vi "Попытка кнопки2.vi"() -> ()   [LabVIEW 2021]
uses:
  <vilib>/Utility/miscctls.llb/LVPositionTypeDef.ctl
  <vilib>/Utility/miscctls.llb/LVBoundsTypeDef.ctl
panel:
  in  "stop":bool
  in  "Вернуть":bool
  out "LED":bool
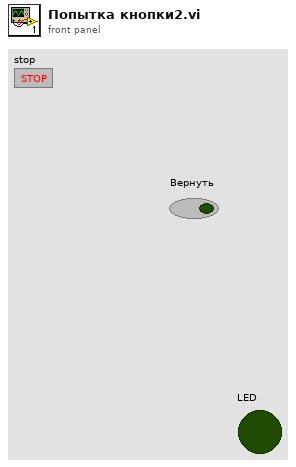
[diagram p1: front panel]
types:
  T1 = typedef "LVPositionTypeDef.ctl" = cluster{"Left":i32, "Top":i32}
  T2 = typedef "LVBoundsTypeDef.ctl" = cluster{"Width":u32, "Height":u32}
  T3 = typedef "LVPoint32TypeDef.ctl" = cluster{"Horizontal":i32, "Vertical":i32}
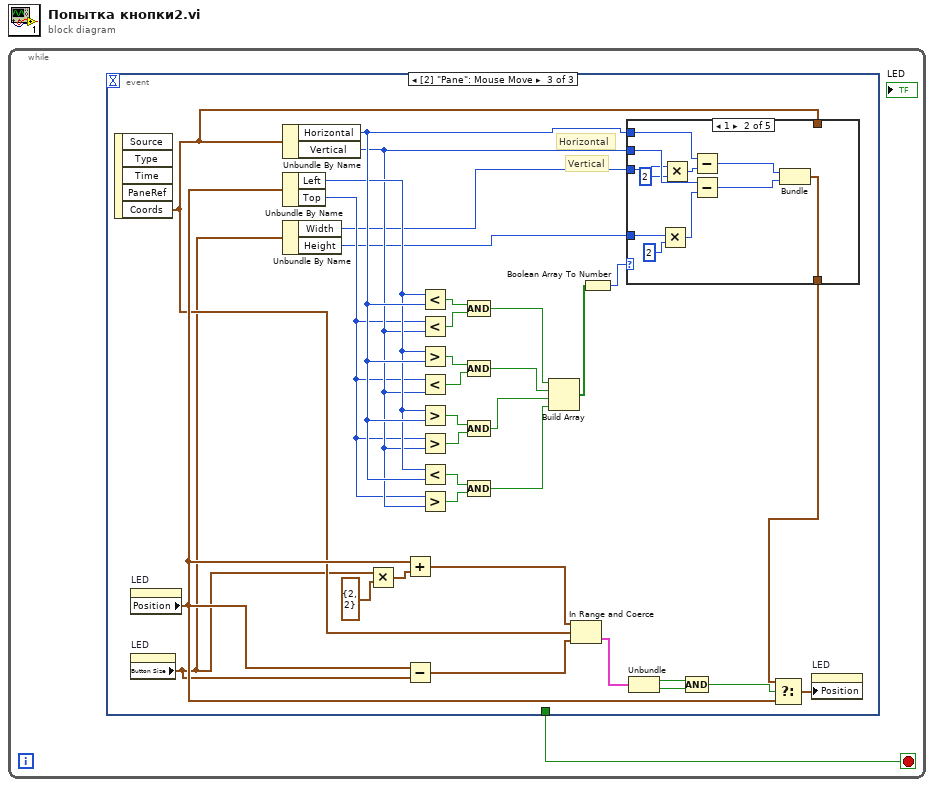
[diagram p0: block diagram]
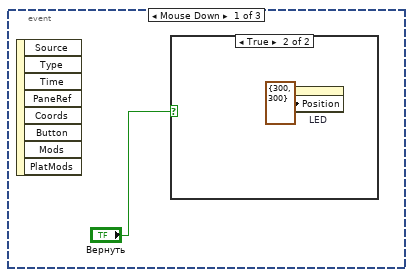
[diagram p2: hidden frame]
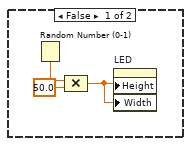
[diagram p3: hidden frame]
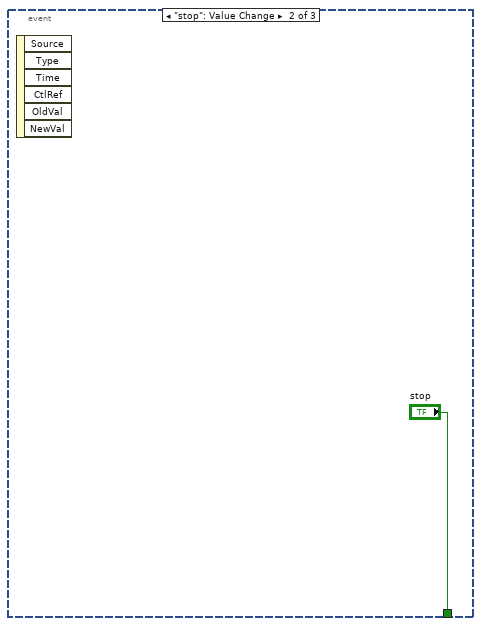
[diagram p4: hidden frame]
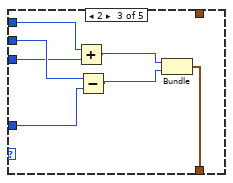
[diagram p6: hidden frame]
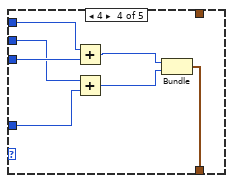
[diagram p7: hidden frame]
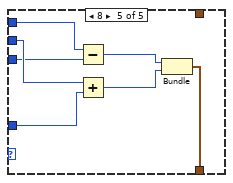
[diagram p8: hidden frame]
diagram:
  n1 = while {
    stop <- w1 stop-if-true
    n2 = event shown="[2] \"Pane\": Mouse Move" {
      selector: _ -> [_ _ _]
      dyn-events: _ -> [_ _ _]
      timeout: _ -> [_ _ _]
      tunnel: [_ "stop" _] -> w1
      event Mouse Down {
        n3 = event-data() -> ()  [unwired: 1 in, 8 out]
        n4 = case shown="True" "Вернуть" {
          frame False {
            n5 = Random Number (0-1)() -> (number: 0 to 1=w5:dbl)
            n6 = Compound Arithmetic op=MULTIPLY(w5, 50.0 ("value")) -> (w4:dbl)
            n7 = property on="LED" class="Bool (strict)"("Height"=w4, "Width"=w4) -> ()  [unwired: 2 in, 2 out]
          }
          frame True {
            n8 = property on="LED" class="Bool (strict)"("Position"=T1 {"Left"=300, "Top"=300}) -> ()  [unwired: 2 in, 2 out]
          }
        }
      }
      event "stop": Value Change {
        n9 = event-data() -> ()  [unwired: 1 in, 6 out]
      }
      event Mouse Move {
        # "Vertical"
        # "Horizontal"
        n10 = event-data() -> ("Coords"=w13:T3)  [unwired: 1 in, 4 out]
        n11 = property on="LED" class="Bool (strict)"() -> ("Position"=w33:T1)  [unwired: 2 in, 2 out]
        n12 = property on="LED" class="Bool (strict)"() -> ("Button Size"=w9:T2)  [unwired: 2 in, 2 out]
        n13 = Unbundle By Name(w13) -> ("Horizontal"=w18:i32, "Vertical"=w16:i32)
        n14 = Unbundle By Name(w33) -> ("Left"=w17:i32, "Top"=w15:i32)
        n15 = Unbundle By Name(w9) -> ("Width"=w12:u32, "Height"=w11:u32)
        n16 = Multiply(x=w9, y=T2 {"Width"=2, "Height"=2}) -> (x*y=w10:T2)
        n17 = Add(x=w33, y=w10) -> (x+y=w34:T2)
        n18 = Subtract(x=w33, y=w9) -> (x-y=w35:T2)
        n19 = Less?(x=w17, y=w18) -> (x < y?=w32:bool)
        n20 = Less?(x=w15, y=w16) -> (x < y?=w31:bool)
        n21 = Greater?(x=w17, y=w18) -> (0:w30:bool)
        n22 = Less?(x=w15, y=w16) -> (x < y?=w29:bool)
        n23 = Greater?(x=w17, y=w18) -> (0:w28:bool)
        n24 = Greater?(x=w15, y=w16) -> (0:w27:bool)
        n25 = Less?(x=w17, y=w18) -> (x < y?=w26:bool)
        n26 = Greater?(x=w15, y=w16) -> (0:w25:bool)
        n27 = Compound Arithmetic op=AND(w32, w31) -> (w24:bool)
        n28 = Compound Arithmetic op=AND(w30, w29) -> (w23:bool)
        n29 = Compound Arithmetic op=AND(w28, w27) -> (w22:bool)
        n30 = Compound Arithmetic op=AND(w26, w25) -> (w21:bool)
        n31 = Build Array(w24, w23, w22, w21) -> (w20:bool[])
        n32 = In Range and Coerce(upper limit=w34, x=w13, lower limit=w35) -> (In Range?=w38:cluster{"Width":bool, "Height":bool})  [unwired: 1 out]
        n33 = Boolean Array To Number(Boolean array=w20) -> (number=w19:u32)
        n34 = case shown="1" w19 {
          tunnel: w18 -> [_ w50 w56 w64 w68]
          tunnel: w12 -> [_ w43 w53 w63 w67]
          tunnel: w16 -> [_ w48 w55 w61 w71]
          tunnel: w11 -> [_ w46 w54 w60 w70]
          tunnel: [w41 w52 w59 w66 w73] -> w14
          tunnel: w13 -> [w41 _ _ _ _]
          frame 0, Default {
          }
          frame 1 {
            n35 = Multiply(x=w46, y=u32 2) -> (x*y=w47:u32)
            n36 = Multiply(x=w43, y=u32 2) -> (x*y=w44:u32)
            n37 = Subtract(x=w50, y=w44) -> (x-y=w51:u32)
            n38 = Subtract(x=w48, y=w47) -> (x-y=w49:u32)
            n39 = Bundle(w51, w49) -> (w52:cluster{u32, u32})  [unwired: 1 in]
          }
          frame 2 {
            n40 = Add(x=w56, y=w53) -> (x+y=w57:u32)
            n41 = Subtract(x=w55, y=w54) -> (x-y=w58:u32)
            n42 = Bundle(w57, w58) -> (w59:cluster{u32, u32})  [unwired: 1 in]
          }
          frame 4 {
            n43 = Add(x=w64, y=w63) -> (x+y=w65:u32)
            n44 = Add(x=w61, y=w60) -> (x+y=w62:u32)
            n45 = Bundle(w65, w62) -> (w66:cluster{u32, u32})  [unwired: 1 in]
          }
          frame 8 {
            n46 = Subtract(x=w68, y=w67) -> (x-y=w69:u32)
            n47 = Add(x=w71, y=w70) -> (x+y=w72:u32)
            n48 = Bundle(w69, w72) -> (w73:cluster{u32, u32})  [unwired: 1 in]
          }
        }
        n49 = Unbundle(w38) -> ("Width"=w37:bool, "Height"=w36:bool)
        n50 = Compound Arithmetic op=AND(w37, w36) -> (w39:bool)
        n51 = Select(t=w14, s=w39, f=w33) -> (s? t:f=w40:cluster{"Horizontal":u32, "Vertical":u32})
        n52 = property on="LED" class="Bool (strict)"("Position"=w40) -> ()  [unwired: 2 in, 2 out]
      }
    }
  }
